vi "Stop Core.vi"(10 "final error code":i32, 11 "GPU FFT Calculator in":refnum<class "GPU FFT Calculator.lvclass">) -> (3 "GPU FFT Calculator out":refnum<class "GPU FFT Calculator.lvclass">)   [LabVIEW 2020, in "GPU FFT Calculator.lvlib" / "GPU FFT Calculator.lvclass"]
doc: "In addition to the following, this method also sends a message to the monitor to notify it that the actor has stopped execution.\n\n(<B>Filename</B>: Actor Framework.lvlib:Actor.lvclass:Stop Core.vi)\n\nDefines what the actor does before it stops. Use the <B>final error code</B> input to determine whether the actor shut down in response to an error.\n\nBy default, this method does nothing. A descendant class may override it to define behavior, such as shutting down any processes the actor initiated in its override of the Actor Core method.\n\nCopyright: MGI\n\nAuthored by Derek Trepanier\nsupport@mooregoodideas.com\nwww.mooregoodideas.com\n\nCopyright (c) 2014, Moore Good Ideas, Inc.\n\nAll rights reserved.\n\nRedistribution and use in source and binary forms, with or without modification, are permitted provided that the following conditions are met:\n\n * Redistributions of source code must retain the above copyright notice, this list of conditions and the following disclaimer.\n * Redistributions in binary form must reproduce the above copyright notice, this list of conditions and the following disclaimer in the documentation and/or other materials provided with the distribution.\n * Neither the name of Moore Good Ideas, Inc. nor the names of its contributors may be used to endorse or promote products derived from this software without specific prior written permission.\n\nTHIS SOFTWARE IS PROVIDED BY THE COPYRIGHT HOLDERS AND CONTRIBUTORS \"AS IS\" AND ANY EXPRESS OR IMPLIED WARRANTIES, INCLUDING, BUT NOT LIMITED TO, THE IMPLIED WARRANTIES OF MERCHANTABILITY AND FITNESS FOR A PARTICULAR PURPOSE ARE DISCLAIMED. IN NO EVENT SHALL THE COPYRIGHT OWNER OR CONTRIBUTORS BE LIABLE FOR ANY DIRECT, INDIRECT, INCIDENTAL, SPECIAL, EXEMPLARY, OR CONSEQUENTIAL DAMAGES (INCLUDING, BUT NOT LIMITED TO, PROCUREMENT OF SUBSTITUTE GOODS OR SERVICES; LOSS OF USE, DATA, OR PROFITS; OR BUSINESS INTERRUPTION) HOWEVER CAUSED AND ON ANY THEORY OF LIABILITY, WHETHER IN CONTRACT, STRICT LIABILITY, OR TORT (INCLUDING NEGLIGENCE OR OTHERWISE) ARISING IN ANY WAY OUT OF THE USE OF THIS SOFTWARE, EVEN IF ADVISED OF THE POSSIBILITY OF SUCH DAMAGE."
uses:
  GPU FFT Calculator.lvclass
  QMH Message.ctl
  GPU FFT Calculator.lvclass/GPU FFT Calculator.ctl
  Calculation Worker/Calculation Worker/Calculation Worker.lvclass
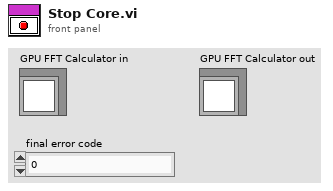
[diagram p1: front panel]
types:
  T1 = typedef "GPU FFT Calculator.lvlib/GPU FFT Calculator.lvclass/QMH Message.ctl" = cluster{"Command":string, "Data":variant}
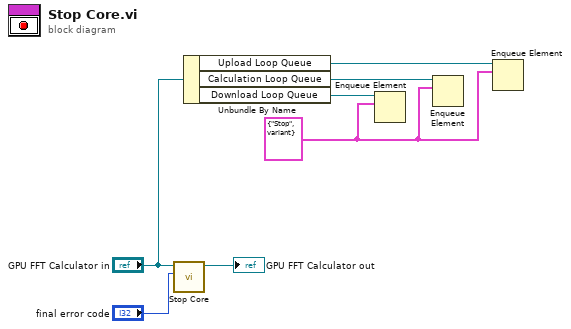
[diagram p0: block diagram]
diagram:
  w1 = T1 {"Command"="Stop", "Data"=variant} ("Cluster")
  n1 = call-parent "Stop Core.vi"("final error code"="final error code", "Calculation Worker in"="GPU FFT Calculator in") -> ("Calculation Worker out"=→"GPU FFT Calculator out":refnum<class "GPU FFT Calculator.lvclass">)  [unwired: 9 in]
  n2 = Unbundle By Name("GPU FFT Calculator in") -> ("Upload Loop Queue"=w2:refnum<queue>, "Calculation Loop Queue"=w3:refnum<queue>, "Download Loop Queue"=w4:refnum<queue>)
  n3 = Enqueue Element(queue=w4, element=w1) -> ()  [unwired: 2 in, 3 out]
  n4 = Enqueue Element(queue=w3, element=w1) -> ()  [unwired: 2 in, 3 out]
  n5 = Enqueue Element(queue=w2, element=w1) -> ()  [unwired: 2 in, 3 out]
